vi "Update Force Calibration Log.vi"(8 "error in (no error)":errorcluster, 9 "array results in":T1, 10 "ia test notifier":refnum<notifier>, 11 "main gui queue":refnum<queue>) -> (0 "error out":errorcluster)   [LabVIEW 2020]
uses:
  Controller Loop/Controller Data.ctl
  Inflation Test/Result Handling/Inflation Test Numeric Results.ctl
  GUI/Main GUI Loop/Handler.ctl
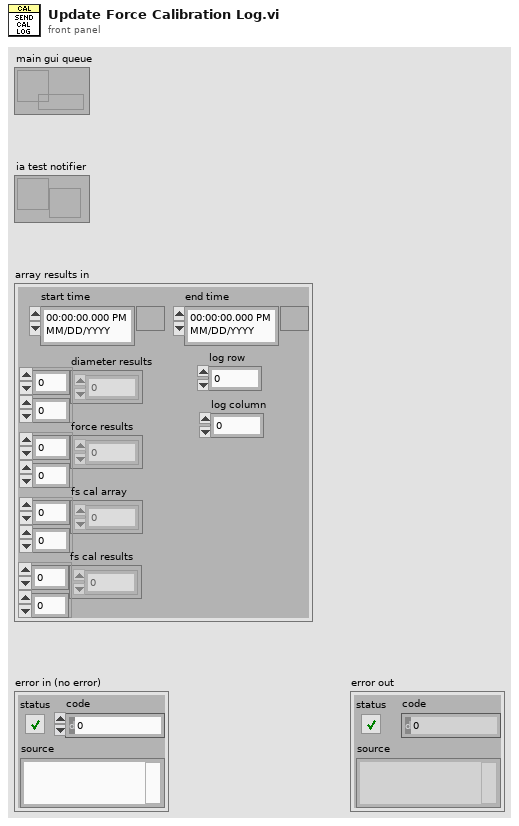
[diagram p1: front panel]
types:
  T1 = typedef "Controller Data.ctl" = cluster{"diameter results":dbl[][], "force results":dbl[][], "fs cal array":dbl[][], "fs cal results":dbl[][], "start time":timestamp, "end time":timestamp, "log row":i32, "log column":i32}
  T2 = typedef "Inflation Test Numeric Results.ctl" = cluster{"diameter":dbl, "diam time":dbl, "force":dbl, "force time":dbl, "setpoint":dbl, "servo pw":dbl, "calibration log":dbl[][], "calibration results":dbl[][]}
  T3 = typedef "Handler.ctl" = cluster{"bool ref":refnum<vi>, "error":errorcluster, "msg":string, "status":string, "switch status":bool, "force cal":dbl[][], "force cal results":dbl[][]}
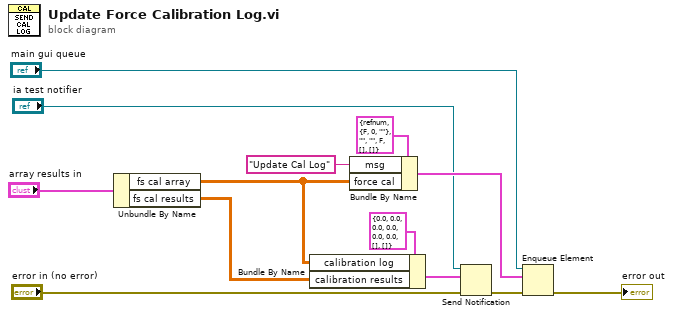
[diagram p0: block diagram]
diagram:
  n1 = Unbundle By Name("array results in") -> ("fs cal array"=w11:dbl[][], "fs cal results"=w12:dbl[][])
  n2 = Bundle By Name(cluster=T2 {"diameter"=0.0, "diam time"=0.0, "force"=0.0, "force time"=0.0, "setpoint"=0.0, "servo pw"=0.0, "calibration log"=[], "calibration results"=[]} ("notification"), "calibration log"=w11, "calibration results"=w12) -> (w8:T2)
  n3 = Bundle By Name(cluster=T3 {"bool ref"=refnum, "error"={"status"=FALSE, "code"=0, "source"=""}, "msg"="", "status"="", "switch status"=FALSE, "force cal"=[], "force cal results"=[]} ("element"), "msg"="Update Cal Log", "force cal"=w11) -> (w10:T3)
  n4 = Send Notification(notification=w8, notifier="ia test notifier", error in (no error)="error in (no error)") -> (error out=w4:errorcluster)  [unwired: 1 out]
  n5 = Enqueue Element(queue="main gui queue", element=w10, error in (no error)=w4) -> (error out=→"error out":errorcluster)  [unwired: 1 in, 2 out]
